vi "CC Observation to Script.vi"(8 "error in (no error)":errorcluster, 11 "Observation":T3={"Priority"=0, "ID"="", "Observer"="", "Obj Name"="", "Obj Type"="", "RA and DEC String"={"RA"="HH:MM:SS.nnn", "DEC"="DEG:arcmin:arcsec.nn"}, "Filter Wheel 1"="", "Filter Wheel 2"="", "Integration Time"=0.0, "Observation Status"=enum."Error", "Offsets"={"RA"=0.0, "DEC"=0.0, "ROT"=0.0}, "Images"=0, "Dither Options"={"Dither"=enum."None", "Dither Radius"=0.0, "Dither Points"=0, "Dither Phase"=0.0}, "Comment 1"="", "Comment 2"=""}) -> (0 "error out":errorcluster, 3 "Script Steps":T1[](array[typedef]))   [LabVIEW 2024]
uses:
  typedefs/CC cluster Observation.ctl
  Observation Queue/CC enum Observation Status.ctl
  Telescope/CC cluster Telescope Offsets.ctl
  typedefs/CC cluster Observation Dither Options.ctl
  typedefs/CC enum Dither Selection.ctl
  typedefs/CC Script Step.ctl
  typedefs/CC enum Script Action.ctl
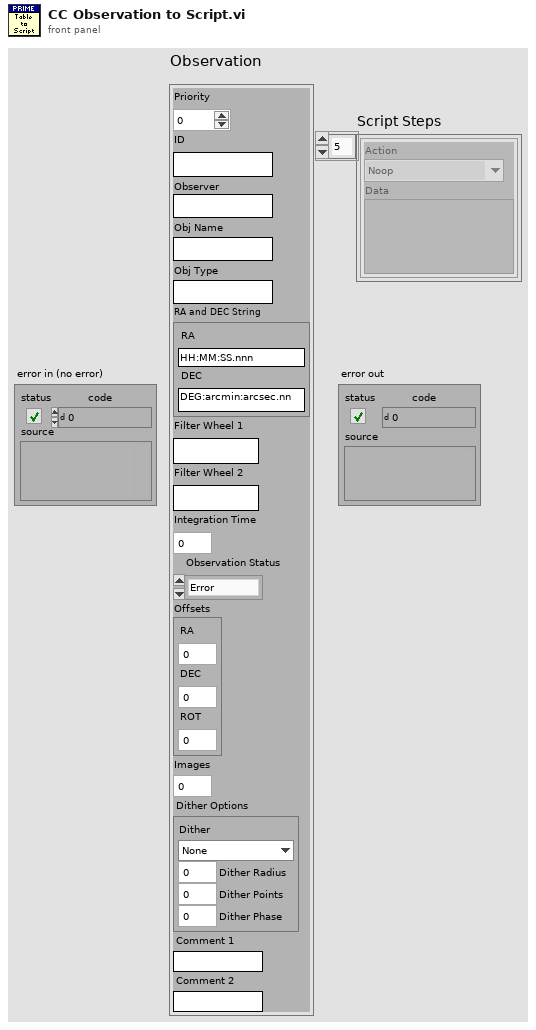
[diagram p1: front panel]
types:
  T1 = typedef "CC Script Step.ctl" = cluster{"Action":T2, "Data":variant}
  T2 = typedef "CC enum Script Action.ctl" = enum16{"Noop", "Define Object", "Define Exposure", "Define Dithering", "Acquire Images", "Set Filter Wheel", "Telescope Home", "Telescope Move", "Telescope RA DEC", "Focus Move Relative", "Focus Move Absolute", "Focus Set Home", "Macro", "Pause", "Ask User", "Define Random Dither"}
  T3 = typedef "CC cluster Observation.ctl" = cluster{"Priority":i32, "ID":string, "Observer":string, "Obj Name":string, "Obj Type":string, "RA and DEC String":cluster{"RA":string, "DEC":string}, "Filter Wheel 1":string, "Filter Wheel 2":string, "Integration Time":dbl, "Observation Status":T4, "Offsets":T5, "Images":i32, "Dither Options":T6, "Comment 1":string, "Comment 2":string}
  T4 = typedef "CC enum Observation Status.ctl" = enum16{"Ready", "Running", "Done", "Error"}
  T5 = typedef "CC cluster Telescope Offsets.ctl" = cluster{"RA":dbl, "DEC":dbl, "ROT":dbl}
  T6 = typedef "CC cluster Observation Dither Options.ctl" = cluster{"Dither":T7, "Dither Radius":dbl, "Dither Points":i32, "Dither Phase":dbl}
  T7 = typedef "CC enum Dither Selection.ctl" = enum16{"None", "Circle", "Random"}
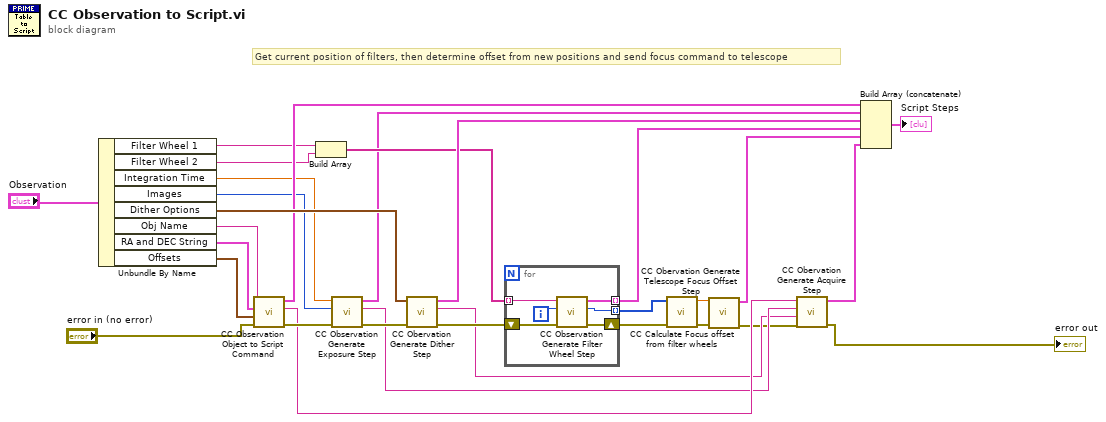
[diagram p0: block diagram]
diagram:
  # "Get current position of filters, then determine offset from new positions and send focus command to telescope"
  n1 = Unbundle By Name("Observation") -> ("Filter Wheel 1"=w25:string, "Filter Wheel 2"=w24:string, "Integration Time"=w21:dbl, "Images"=w7:i32, "Dither Options"=w27:T6, "Obj Name"=w17:string, "RA and DEC String"=w18:cluster{"RA":string, "DEC":string}, "Offsets"=w19:T5)
  n2 = call "CC Observation Object to Script Command.vi"("error in (no error)"="error in (no error)", "Offsets"=w19, "RA and DEC String"=w18, "Object.Name"=w17) -> ("error out"=w16:errorcluster, "Object Name out"=w10:string, "Define Object Step"=w26:T1)  [unwired: 5 in]
  n3 = Build Array(w25, w24) -> (w23:string[])
  n4 = call "CC Observation Generate Exposure Step.vi"("error in (no error)"=w16, "Images"=w7, "Integration Time"=w21) -> ("error out"=w15:errorcluster, "Exp Name"=w9:string, "Exp Step"=w20:T1)  [unwired: 6 in]
  n5 = call "CC Obervation Generate Dither Step.vi"("error in (no error)"=w15, "Dither Options"=w27) -> ("error out"=w14:errorcluster, "Name"=w8:string, "Step"=w28:T1)  [unwired: 7 in]
  n6 = for {
    tunnel: w23 -> [w36] mode=indexing
    tunnel: [w34] -> w22 mode=indexing
    shift-right: [w32] -> w6
    shift-left: w14 -> [w33]
    tunnel: [w31] -> w5 mode=indexing
    i -> [w35]
    n7 = call "CC Observation Generate Filter Wheel Step.vi"("error in (no error)"=w33, "Wheel (0 or 1)"=w35, "Filter Wheel Name"=w36) -> ("error out"=w32:errorcluster, "filter idx"=w31:i32, "Step"=w34:T1)  [unwired: 6 in]
  }
  n8 = call "CC Calculate Focus offset from filter wheels.vi"("error in (no error)"=w6, "Filter positions"=w5) -> ("error out"=w3:errorcluster, "New focus offset"=w4:dbl)  [unwired: 8 in]
  n9 = call "CC Obervation Generate Telescope Focus Offset Step.vi"("error in (no error)"=w3, "Offset"=w4) -> ("error out"=w2:errorcluster, "Steps"=w1:T1[])  [unwired: 8 in]
  n10 = call "CC Obervation Generate Acquire Step.vi"("error in (no error)"=w2, "Dithering"=w8, "Exposure"=w9, "Object"=w10) -> ("error out"=→"error out":errorcluster, "Acquire Step"=w11:T1)  [unwired: 6 in]
  n11 = Build Array (concatenate)(w26, w20, w28, w22, w1, w11) -> (→"Script Steps":T1[])
